vi "UFO Shadow Launcher.vi"(8 "error in (no error)":errorcluster) -> (0 "error out":errorcluster, 3 "Command Queue":refnum<queue>)   [LabVIEW 2019]
doc: "Sets up the UFO shadow VI and starts it asynchronously. The command queue for the window is returned."
uses:
  Slave Window Command Message.ctl
  Slave Window Command.ctl
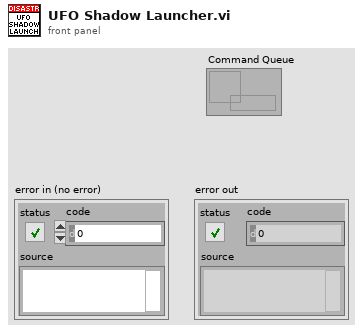
[diagram p1: front panel]
types:
  T1 = typedef "Slave Window Command Message.ctl" = cluster{"Command":T2, "Data":variant}
  T2 = typedef "Slave Window Command.ctl" = enum16{"Open", "Set Bounds", "Set Opacity", "Close", "Frame"}
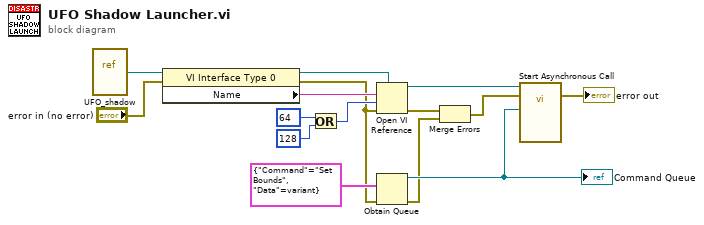
[diagram p0: block diagram]
diagram:
  n1 = vi-ref "UFO_shadow.vi"() -> (w14:refnum<vi>)
  n2 = property class="VI Interface Type 0"(reference=w14, error in="error in (no error)") -> (reference out=w12:refnum<vi>, error out=w5:errorcluster, "Name"=w13:string)
  n3 = Or(x=64 ("options"), y=128 ("options")) -> (x .or. y?=w9:i32)
  n4 = Open VI Reference(type specifier VI Refnum (for type only)=w12, vi path=w13, options=w9, error in (no error)=w5) -> (vi reference=w8:refnum<vi>, error out=w4:errorcluster)  [unwired: 2 in]
  n5 = Obtain Queue(element data type=T1 {"Command"=enum."Set Bounds", "Data"=variant} ("Command Message"), error in (no error)=w5) -> (queue out=w7:refnum<queue>, error out=w3:errorcluster)  [unwired: 3 in, 1 out]
  "Command Queue" <- w7
  n6 = Merge Errors(w4, w3) -> (w2:errorcluster)
  n7 = call-by-ref "Start Asynchronous Call"(reference=w8, error in=w2, "Command Queue"=w7) -> (error out=→"error out":errorcluster)  [unwired: 11 in, 1 out]
